vi "Determine Clothoid Values.vi"(10 "Scaling":dbl, 11 "Desired Length":dbl) -> (0 "Center Point":cluster{dbl, dbl}, 1 "Tangent Angle rad":dbl, 2 "Para Time":dbl, 3 "Vertex Dist ft":dbl)   [LabVIEW 2020]
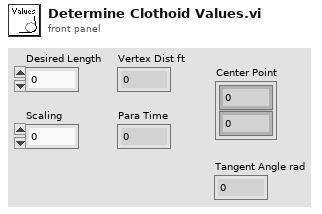
[diagram p1: front panel]
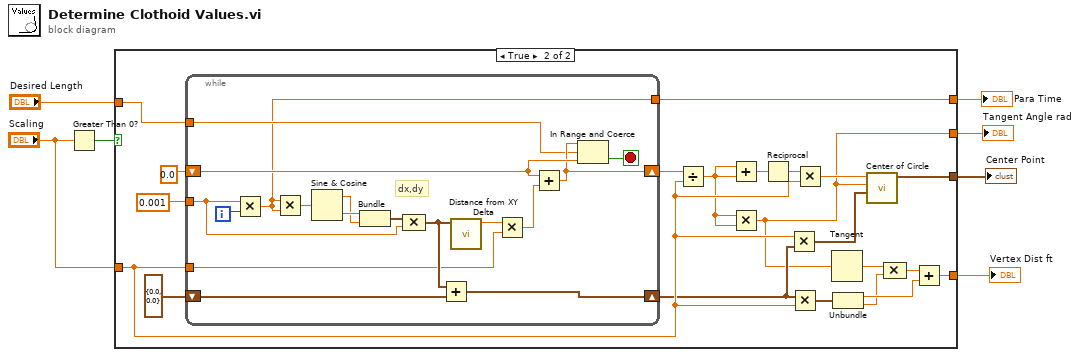
[diagram p0: block diagram]
diagram:
  n1 = Greater Than 0?(x="Scaling") -> (x > 0?=w5:bool)
  n2 = case shown="True" w5 {
    tunnel: "Scaling" -> [_ w12]
    tunnel: [_ w21] -> w7
    tunnel: "Desired Length" -> [_ w19]
    tunnel: [_ w18] -> w3
    tunnel: [_ w13] -> w2
    tunnel: [_ w8] -> w1
    frame False {
    }
    frame True {
      n3 = while {
        shift-right: [w35] -> w11
        shift-left: cluster{dbl, dbl} {0.0, 0.0} -> [w40]
        tunnel: 0.001 -> [w39]
        shift-right: [w37] -> w15
        shift-left: 0.0 -> [w38]
        tunnel: w12 -> [w29]
        tunnel: w19 -> [w33]
        tunnel: [w32] -> w18
        i -> [w45]
        stop <- w36 stop-if-true
        # "dx,dy"
        n4 = Multiply(x=w39, y=w45) -> (x*y=w32:dbl)
        n5 = Multiply(x=w32, y=w32) -> (x*y=w44:dbl)
        n6 = Sine & Cosine(0:w44) -> (1:w42:dbl, 2:w43:dbl)
        n7 = Bundle(w43, w42) -> (w41:cluster{dbl, dbl})  [unwired: 1 in]
        n8 = Compound Arithmetic op=MULTIPLY(w41, w39) -> (w31:cluster{dbl, dbl})
        n9 = Add(x=w31, y=w40) -> (x+y=w35:cluster{dbl, dbl})
        n10 = call "Distance from XY Delta.vi"("Delta Point"=w31) -> ("Distance"=w30:dbl)  [unwired: 10 in]
        n11 = Multiply(x=w30, y=w29) -> (x*y=w34:dbl)
        n12 = Add(x=w38, y=w34) -> (x+y=w37:dbl)
        n13 = In Range and Coerce(upper limit=w37, x=w33, lower limit=w38) -> (In Range?=w36:bool)  [unwired: 1 out]
      }
      n14 = Divide(x=w15, y=w12) -> (x/y=w9:dbl)
      n15 = Add(x=w9, y=w9) -> (x+y=w17:dbl)
      n16 = Multiply(x=w9, y=w9) -> (x*y=w8:dbl)
      n17 = Reciprocal(x=w17) -> (1/x=w16:dbl)
      n18 = Multiply(x=w12, y=w11) -> (x*y=w10:cluster{dbl, dbl})
      n19 = Multiply(x=w11, y=w12) -> (x*y=w20:cluster{dbl, dbl})
      n20 = Multiply(x=w16, y=w12) -> (x*y=w14:dbl)
      n21 = Tangent(1:w8) -> (0:w22:dbl)
      n22 = Unbundle(w20) -> (w25:dbl, w23:dbl)
      n23 = call "Center of Circle.vi"("Tangent Point"=w10, "Tangent Angle"=w8, "Radius"=w14) -> ("Center Point"=w13:cluster{dbl, dbl})  [unwired: 8 in]
      n24 = Compound Arithmetic op=MULTIPLY(w22, w23) -> (w24:dbl)
      n25 = Add(x=w24, y=w25) -> (x+y=w21:dbl)
    }
  }
  "Vertex Dist ft" <- w7
  "Para Time" <- w3
  "Center Point" <- w2
  "Tangent Angle rad" <- w1
